vi "channel scaling class trial.vi"() -> ()   [LabVIEW 2018]
uses:
  RT/Type Defs/channelScalingTypes.ctl
  RT/Type Defs/scalingMethods.ctl
  RT/Type Defs/channelCalibration.ctl
panel:
  in  "Data received":sgl[][](array[numeric])=array62x1849[114638 elements]
  out "Table Control":string[][](table)
  out "scaled data":sgl[][](array[numeric])
  out "Array":T1[](array[typedef])
  in  "file path (use dialog)":path
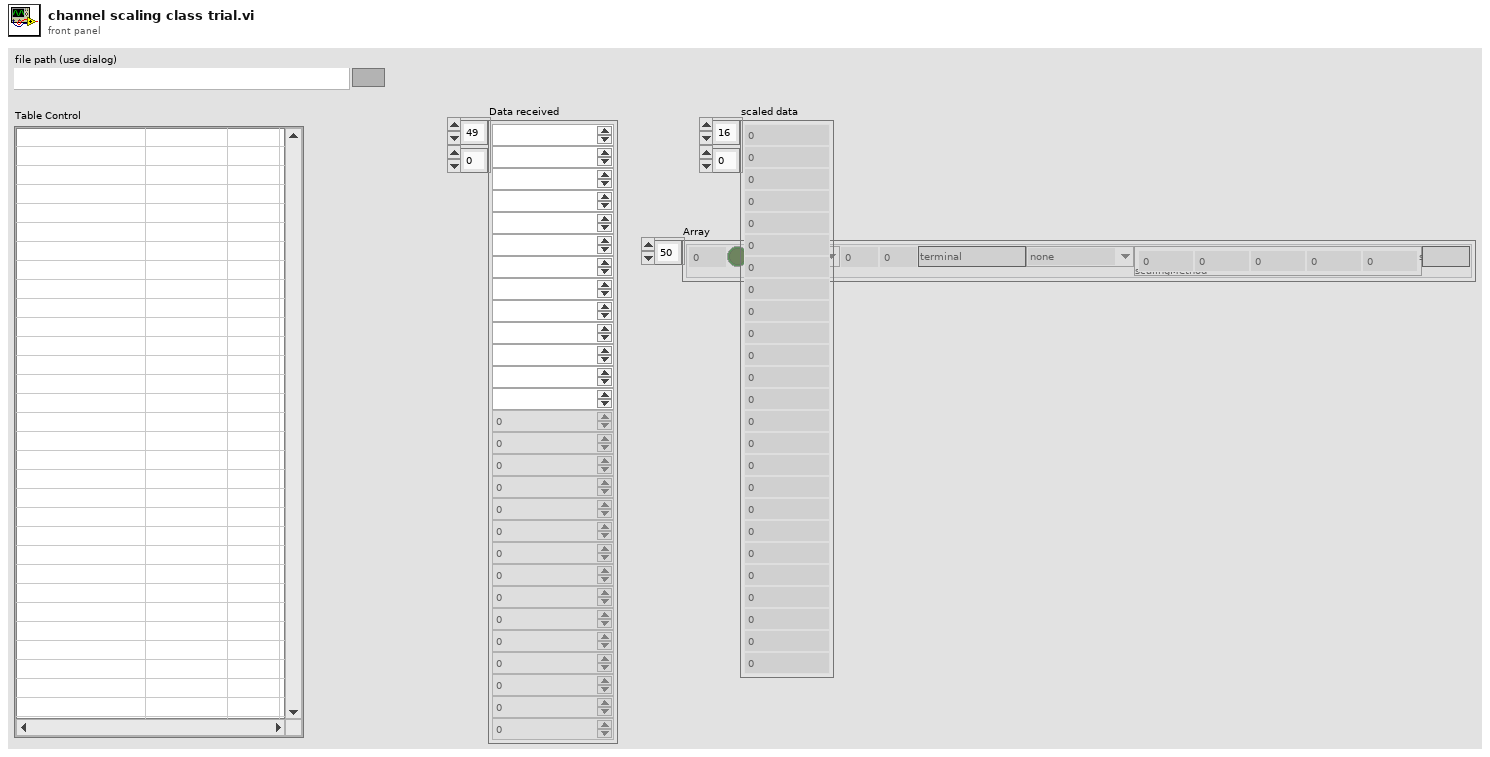
[diagram p1: front panel]
types:
  T1 = typedef "channelCalibration.ctl" = cluster{"index":u16, "active":bool, "channelType":T2, "module":u16, "terminal":u16, "channelName":string, "scalingMethod":T3, "scalingParameters":dbl[], "scaledUnits":string}
  T2 = typedef "channelScalingTypes.ctl" = enum16{"calculation", "measurement", "scanivalve", "output", "digital"}
  T3 = typedef "scalingMethods.ctl" = enum16{"none", "linear", "thermocouple", "polynomial", "encoder", "RTD"}
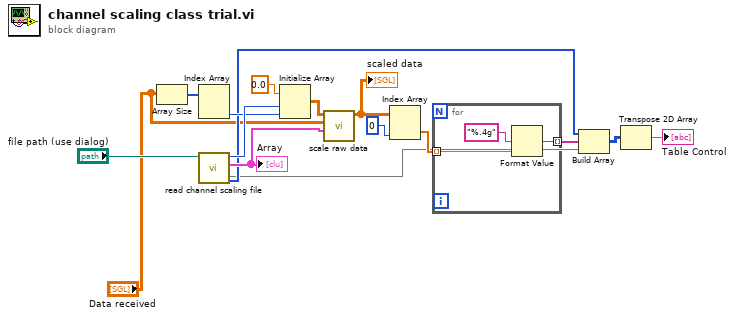
[diagram p0: block diagram]
diagram:
  n1 = Array Size(array="Data received") -> (size(s)=w13:i32[])
  n2 = Index Array(array=w13) -> (element #2=w12:i32)  [unwired: 2 in, 1 out]
  n3 = call "read channel scaling file.vi"("file path"="file path (use dialog)") -> ("channelTypeCount"=w7:i32[], "channelConfig"=w15:T1[], "activeChannelCount"=w14:u16, 4:w2)  [unwired: 5 in, 2 out]
  "Array" <- w15
  n4 = Initialize Array(sgl 0.0 ("Numeric"), w14, w12) -> (w10:sgl[][])
  n5 = call "scale raw data.vi"("channelScaling"=w15, "raw data"="Data received", "scaled data"=w10) -> ("scaled data"=w9:dbl[][])  [unwired: 8 in]
  "scaled data" <- w9
  n6 = Index Array(array=w9, index (col)=0 ("disabled index (col)")) -> (element=w8:dbl[])  [unwired: 1 in]
  n7 = for {
    tunnel: w8 -> [w19] mode=indexing
    tunnel: [w17] -> w6 mode=indexing
    n8 = Format Value(format string="%.4g", value (0)=w19) -> (output string=w17:string)  [unwired: 1 in]
  }
  n9 = Build Array(w7, w6, w2) -> (w4:i32[][])
  n10 = Transpose 2D Array(2D array=w4) -> (transposed array=→"Table Control":i32[][])
